vi "fgv_global-stop.vi"(7 "cmd":enum16{"init", "stop", "read"}(ring)) -> (3 "val_out":bool)   [LabVIEW 2019]
uses:
  Ctrl/cmd_ini-RW.ctl
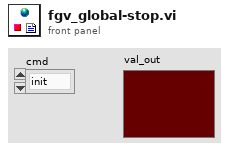
[diagram p1: front panel]
types:
  T1 = cluster{"Ntrip tcp":bool, "GNSS serial":bool, "RTCM serial":bool, "Extra serial":bool}
  T2 = typedef "cmd_ini-RW.ctl" = enum16{"ini", "read", "write"}
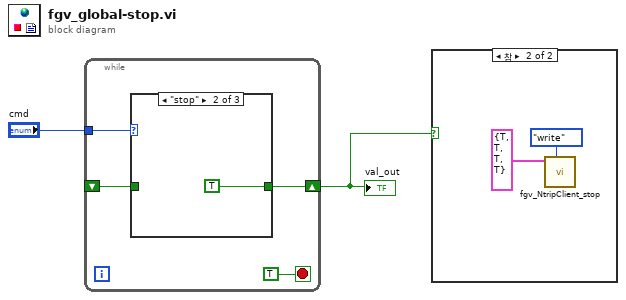
[diagram p0: block diagram]
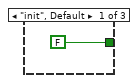
[diagram p3: hidden frame]
diagram:
  n1 = while {
    tunnel: "cmd" -> [w5]
    shift-right: [w4] -> w1
    shift-left: _ -> [w3]
    stop <- TRUE stop-if-true
    n2 = case shown="\"stop\"" w5 {
      tunnel: [FALSE TRUE w9] -> w4
      tunnel: w3 -> [_ _ w9]
      frame "init", Default {
      }
      frame "stop" {
      }
      frame "read" {
      }
    }
  }
  "val_out" <- w1
  n3 = case shown="참" w1 {
    frame False {
    }
    frame True {
      n4 = call "fgv_NtripClient_stop.vi"("cmd"=cmd_ini-RW."write", "local stops"=T1 {"Ntrip tcp"=TRUE, "GNSS serial"=TRUE, "RTCM serial"=TRUE, "Extra serial"=TRUE}) -> ()  [unwired: 9 in, 1 out]
    }
  }
